vi "read_params.vi"(8 "error in (no error)":errorcluster, 11 "NuSVC in":refnum<class "NuSVC.lvclass">) -> (0 "error out":errorcluster, 2 "params":T1={"nu"=0.5, "kernel"="rbf", "degree"=3.0, "gamma"={"gamma_type"="scale", "gamma_float"=0.001}, "coef0"=0.0, "shrinking"=TRUE, "probability"=FALSE, "tol"=0.001, "cache_size"=200.0, "class_weight"={"class_weight_type"="None", "class_weight_dict"="{0:1.2,1:0.8,2:1.0}"}, "verbose"=FALSE, "max_iter"=-1.0, "decision_function_shape"="ovr", "break_ties"=FALSE, "random_state"=0.0}, 3 "NuSVC out":refnum<class "NuSVC.lvclass">)   [LabVIEW 2020, in "NuSVC.lvclass"]
uses:
  NuSVC.lvclass
  Controls/nu_svc_params.ctl
  NuSVC.lvclass/NuSVC.ctl
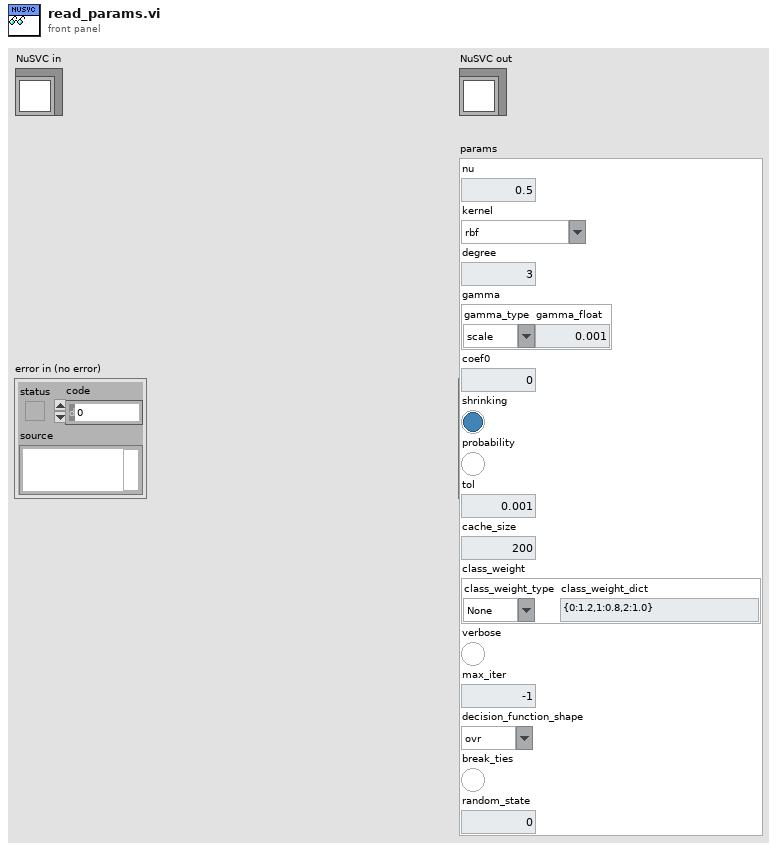
[diagram p1: front panel]
types:
  T1 = typedef "nu_svc_params.ctl" = cluster{"nu":dbl, "kernel":string, "degree":dbl, "gamma":cluster{"gamma_type":string, "gamma_float":dbl}, "coef0":dbl, "shrinking":bool, "probability":bool, "tol":dbl, "cache_size":dbl, "class_weight":cluster{"class_weight_type":string, "class_weight_dict":string}, "verbose":bool, "max_iter":dbl, "decision_function_shape":string, "break_ties":bool, "random_state":dbl}
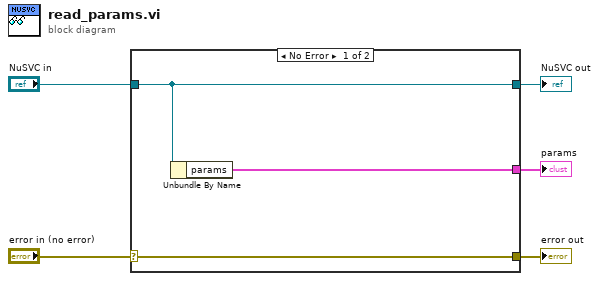
[diagram p0: block diagram]
diagram:
  n1 = case shown="No Error" "error in (no error)" {
    selector: "error in (no error)" -> [w8 w9]
    tunnel: [w8 w9] -> w4
    tunnel: [w7 w10] -> w2
    tunnel: "NuSVC in" -> [w7 w10]
    tunnel: [w6 _] -> w1
    frame No Error {
      n2 = Unbundle By Name(w7) -> ("params"=w6:T1)
    }
    frame Error {
    }
  }
  "error out" <- w4
  "NuSVC out" <- w2
  "params" <- w1
